vi "Read Arg.vi"(0 "class data in":refnum<class "MB_ENGINE.lvclass">, 11 "error in (no error)":errorcluster) -> (4 "class data out":refnum<class "MB_ENGINE.lvclass">, 6 "02":u16, 8 "03":u16, 15 "error out":errorcluster)   [LabVIEW 2019, in "MB_ENGINE.lvclass"]
uses:
  MB_ENGINE.lvclass
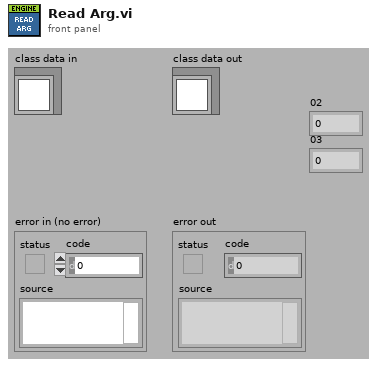
[diagram p1: front panel]
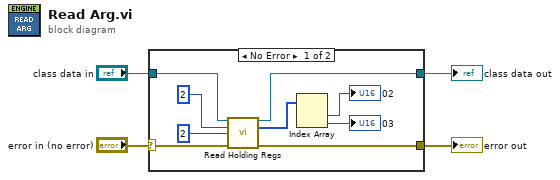
[diagram p0: block diagram]
diagram:
  n1 = case shown="No Error" "error in (no error)" {
    selector: "error in (no error)" -> [w12 w15]
    tunnel: [w11 w15] -> w3
    tunnel: "class data in" -> [w13 w14]
    tunnel: [w5 w14] -> w1
    frame No Error {
      n2 = call-dynamic "Read Holding Regs.vi"("reference in"=w13, "starting address"=u16 2, "number of inputs"=u16 2, "error in (no error)"=w12) -> ("reference out"=w5:refnum<class "MB_ENGINE.lvclass">, "register values"=w6:u16[], "error out"=w11:errorcluster)  [unwired: 9 in]
      n3 = Index Array(array=w6) -> (element #1=→"02":u16, element #2=→"03":u16)  [unwired: 2 in]
    }
    frame Error {
    }
  }
  "error out" <- w3
  "class data out" <- w1
